vi "GetTimingGrpInfo.vi"(8 "error in":errorcluster, 11 "TimingGrp in":refnum<class "TimingGrp.lvclass">) -> (0 "error out":errorcluster, 1 "Num of Chans":i32, 2 "Multi Rate Mods in Timing Grp":T2, 3 "All TimingGrp Chans":string[](array[string]), 4 "Timing Cfg":T1, 6 "Grp List":string[][](array[string]))   [LabVIEW 2012, in "Configuration Grandmaster.lvlib" / "TimingGrp.lvclass"]
uses:
  TimingGrp.lvclass
  SubVIs Main/SubVIs Build Grp/Custom Ctrls Bld/ge_MultiRateMods.ctl
  Common/Controls/Group Timing Info.ctl
  TimingGrp.lvclass/TimingGrp.ctl
  Class Chan Group/Read GrpName.vi
  Class Chan Group/Read MeasType.vi
  Class Chan Group/ChanGrp.lvclass
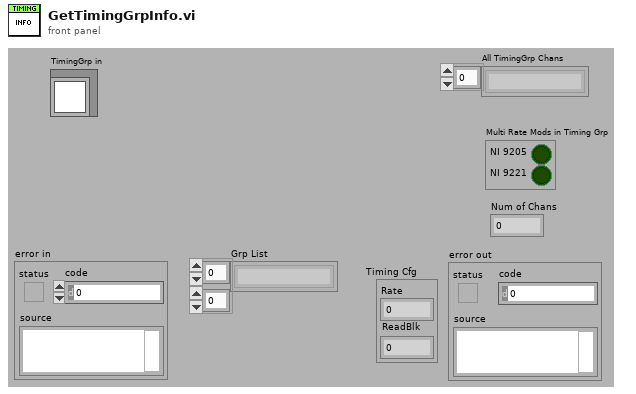
[diagram p1: front panel]
types:
  T1 = typedef "Group Timing Info.ctl" = cluster{"Rate":dbl, "ReadBlk":i32}
  T2 = typedef "ge_MultiRateMods.ctl" = cluster{"NI 9205":bool, "NI 9221":bool}
  T3 = typedef "ge_MeasType.ctl" = enum16{"Voltage", "Frequency", "Tachometer", "Dynamic", "Thermocouple", "RTD", "Strain", "Current", "Resistance"}
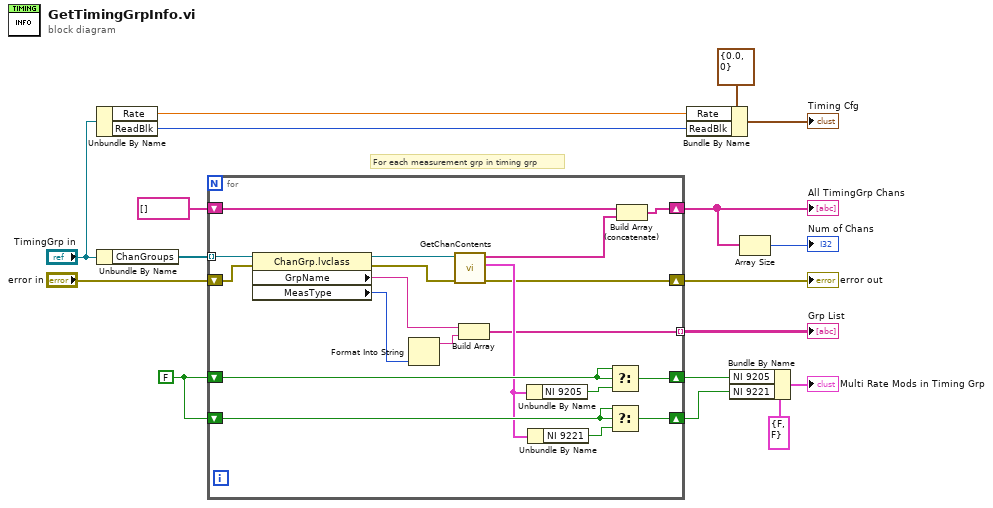
[diagram p0: block diagram]
diagram:
  w17 = FALSE
  # "For each measurement grp in timing grp"
  n1 = Unbundle By Name("TimingGrp in") -> ("Rate"=w3:dbl, "ReadBlk"=w2:i32)
  n2 = Unbundle By Name("TimingGrp in") -> ("ChanGroups"=w9:refnum<class "ChanGrp.lvclass">[])
  n3 = for {
    shift-right: [w34] -> w15
    shift-left: w17 -> [w36]
    shift-right: [w31] -> w14
    shift-left: w17 -> [w33]
    shift-right: [w29] -> w10
    shift-left: string[] [] ("Grp Chans") -> [w30]
    tunnel: w9 -> [w25] mode=indexing
    shift-right: [w26] -> w7
    shift-left: "error in" -> [w22]
    tunnel: [w18] -> w1 mode=indexing
    n4 = property class="ChanGrp.lvclass"(reference=w25, error in=w22) -> (reference out=w24:refnum<class "ChanGrp.lvclass">, error out=w23:errorcluster, "GrpName"=w20:string, "MeasType"=w19:T3)
    n5 = Format Into String(w19) -> (resulting string=w21:string)  [unwired: 3 in, 1 out]
    n6 = call "GetChanContents.vi"("error in"=w23, "ChanGrp.lvclass"=w24) -> ("error out"=w26:errorcluster, "Multi Rate Mods in Grp"=w28:T2, "All GrpChan Names"=w27:string[])  [unwired: 3 in, 4 out]
    n7 = Build Array(w20, w21) -> (w18:string[])
    n8 = Unbundle By Name(w28) -> ("NI 9205"=w35:bool)
    n9 = Unbundle By Name(w28) -> ("NI 9221"=w32:bool)
    n10 = Select(t=w36, s=w36, f=w35) -> (s? t:f=w34:bool)
    n11 = Select(t=w33, s=w33, f=w32) -> (s? t:f=w31:bool)
    n12 = Build Array (concatenate)(w30, w27) -> (w29:string[])
  }
  "All TimingGrp Chans" <- w10
  "error out" <- w7
  "Grp List" <- w1
  n13 = Bundle By Name(cluster=T1 {"Rate"=0.0, "ReadBlk"=0} ("Timing Cfg"), "Rate"=w3, "ReadBlk"=w2) -> (→"Timing Cfg":T1)
  n14 = Bundle By Name(cluster=T2 {"NI 9205"=FALSE, "NI 9221"=FALSE} ("Multi Rate Mods in Grp"), "NI 9205"=w15, "NI 9221"=w14) -> (→"Multi Rate Mods in Timing Grp":T2)
  n15 = Array Size(array=w10) -> (size(s)=→"Num of Chans":i32)
